vi "weightSerialRead_LoadCell_S.vi"(1 "Serial Settings":T1={"baud rate"=9600, "data bits"=8, "parity"=enum."None", "stop bits"=10, "flow control"=0} {"flow control" items=["None"=0, "XON/XOFF"=1, "RTS/CTS"=2, "DTR/DSR"=4]; "stop bits" items=["1.0"=10, "1.5"=15, "2.0"=20]; "data bits" min=5 max=8 step=1; "baud rate" items=["75"=75, "110"=110, "134"=134, "150"=150, "300"=300, "600"=600, "1200"=1200, "1800"=1800, "2400"=2400, "4800"=4800, "7200"=7200, "9600"=9600, "14400"=14400, "19200"=19200, "28800"=28800, "38400"=38400, "56000"=56000, "57600"=57600, "115200"=115200, "128000"=128000, "230400"=230400]}, 2 "Weight VISA resource name":refnum<visa-resource-name>="COM1", 3 "delay before read (ms)":u32=500) -> (0 "String":string)   [LabVIEW 2019]
doc: "Serial read one time of the weight (flipped the weight because the weighing balance reads reversed weights)"
uses:
  Program Files (x86)/National Instruments/LabVIEW 2019/examples/Instrument IO/Serial/support/Serial - Settings.ctl
  <vilib>/Instr/_visa.llb/VISA Configure Serial Port (Instr).vi
panel:
  out "bytes read":u32
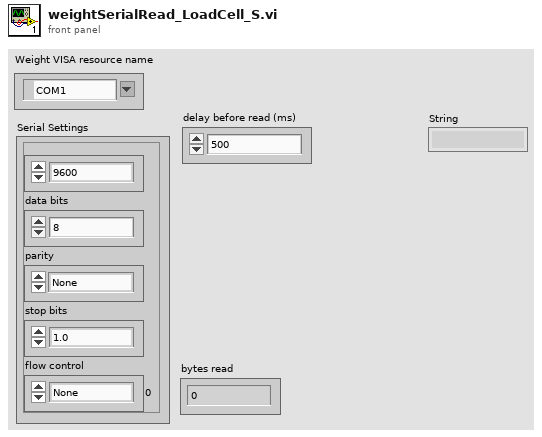
[diagram p1: front panel]
types:
  T1 = typedef "Serial - Settings.ctl" = cluster{"baud rate":u32, "data bits":u16, "parity":enum16{"None", "Odd", "Even", "Mark", "Space"}, "stop bits":u16, "flow control":u16}
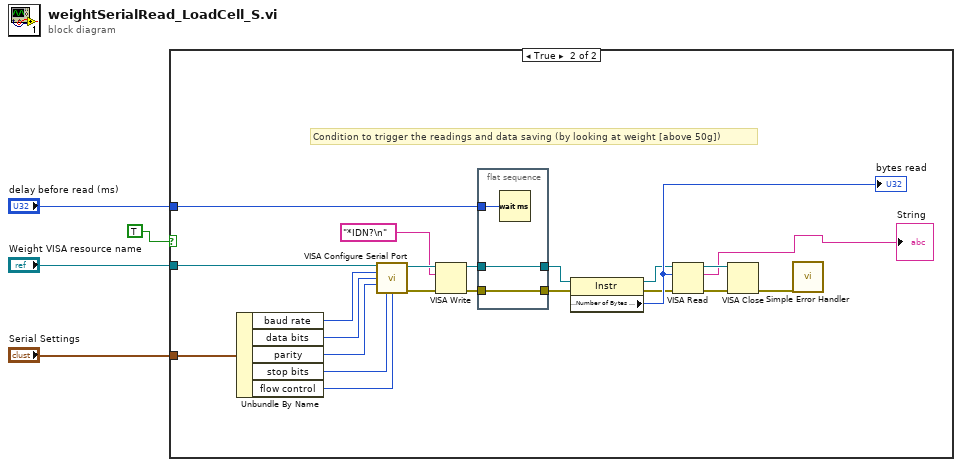
[diagram p0: block diagram]
diagram:
  n1 = case shown="True" TRUE {
    tunnel: "Serial Settings" -> [_ w21]
    tunnel: "delay before read (ms)" -> [_ w17]
    tunnel: "Weight VISA resource name" -> [_ w7]
    frame False {
    }
    frame True {
      # "Condition to trigger the readings and data saving (by looking at weight [above 50g])"
      n2 = Unbundle By Name(w21) -> ("baud rate"=w22:u32, "data bits"=w23:u16, "parity"=w24:enum16{"None", "Odd", "Even", "Mark", "Space"}, "stop bits"=w25:u16, "flow control"=w26:u16)
      n3 = call-poly "VISA Configure Serial Port"("VISA resource name"=w7, "baud rate (9600)"=w22, "data bits (8)"=w23, "parity (0:none)"=w24, "stop bits (10: 1 bit)"=w25, "flow control (0:none)"=w26) -> ("VISA resource name out"=w9:refnum<visa-resource-name>, "error out"=w8:errorcluster)  [unwired: 3 in, 5 out]
      n4 = VISA Write(VISA resource name=w9, write buffer="*IDN?\n" ("Command"), error in (no error)=w8) -> (VISA resource name out=w15:refnum<visa-resource-name>, error out=w13:errorcluster)  [unwired: 1 out]
      n5 = flat-sequence {
        tunnel: w13 -> [w28]
        tunnel: [w28] -> w14
        tunnel: w15 -> [w27]
        tunnel: [w27] -> w16
        tunnel: w17 -> [w29]
        frame #0 {
          n6 = Wait (ms)(milliseconds to wait=w29) -> ()  [unwired: 1 out]
        }
      }
      n7 = property class="Instr"(reference=w16, error in=w14) -> (reference out=w18:refnum<visa-resource-name>, error out=w19:errorcluster, "Serial Settings:Number of Bytes at Serial Port"=w20:u32)
      "bytes read" <- w20
      n8 = VISA Read(VISA resource name=w18, byte count=w20, error in (no error)=w19) -> (VISA resource name out=w11:refnum<visa-resource-name>, read buffer=→"String":string, error out=w10:errorcluster)  [unwired: 1 out]
      n9 = VISA Close(VISA resource name=w11, error in (no error)=w10) -> (error out=w12:errorcluster)
      n10 = call <vilib>:"Simple Error Handler.vi"("error in (no error)"=w12) -> ()  [unwired: 1 in, 8 out]
    }
  }
